vi "RevertVMs.vi"(8 "error in (no error)":errorcluster, 10 "Array":bool[](array[boolean])=[TRUE, TRUE, TRUE, TRUE, TRUE, TRUE, TRUE, TRUE]) -> (0 "error out":errorcluster)   [LabVIEW 2013]
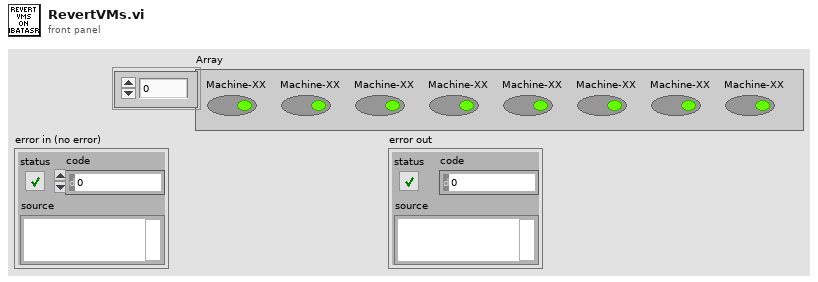
[diagram p1: front panel]
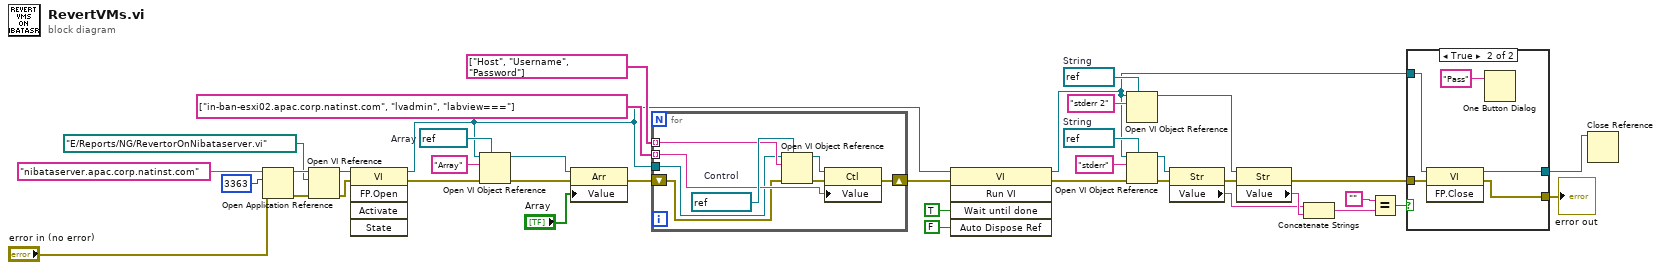
[diagram p0: block diagram]
diagram:
  w18 = refnum<vi> refnum  # String
  w23 = refnum<vi> refnum  # String
  w34 = refnum<vi> refnum  # Array
  n1 = Open Application Reference(8:"error in (no error)", 10:u16 3363 ("port number or service name (3363)"), 11:"nibataserver.apac.corp.natinst.com" ("machine name (\"\":  open local reference)")) -> (0:w37:errorcluster, 3:w36:refnum<vi>)  [unwired: 1 in]
  n2 = Open VI Reference(application reference (local)=w36, vi path=path "E:/Reports/NG/RevertorOnNibataserver.vi", error in (no error)=w37) -> (vi reference=w35:refnum<vi>, error out=w4:errorcluster)  [unwired: 3 in]
  n3 = invoke class="VI" method="FP.Open"(reference=w35, error in=w4) -> (reference out=w6:refnum<vi>, error out=w7:errorcluster)  [unwired: 3 in, 3 out]
  n4 = Open VI Object Reference(7:w34, 8:w7, 10:"Array" ("Text.Text"), 11:w6) -> (0:w32:errorcluster, 3:w33:refnum<vi>)
  n5 = property class="Arr"(reference=w33, error in=w32, "Value"="Array") -> (error out=w26:errorcluster)  [unwired: 1 out]
  n6 = for {
    tunnel: string[] ["Host", "Username", "Password"] -> [w45] mode=indexing
    tunnel: string[] ["in-ban-esxi02.apac.corp.natinst.com", "lvadmin", "labview==="] -> [w44] mode=indexing
    shift-right: [w42] -> w12
    shift-left: w26 -> [w41]
    tunnel: w6 -> [w40]
    w47 = refnum<vi> refnum  # Control
    n7 = Open VI Object Reference(7:w47, 8:w41, 10:w45, 11:w40) -> (0:w43:errorcluster, 3:w46:refnum<vi>)
    n8 = property class="Ctl"(reference=w46, error in=w43, "Value"=w44) -> (error out=w42:errorcluster)  [unwired: 1 out]
  }
  n9 = invoke class="VI" method="Run VI"(reference=w6, error in=w12, "Wait until done"=TRUE ("Wait Until Done"), "Auto Dispose Ref"=FALSE ("Auto Dispose Reference")) -> (reference out=w5:refnum<vi>, error out=w11:errorcluster)  [unwired: 1 in, 3 out]
  n10 = Open VI Object Reference(7:w18, 10:"stderr 2" ("name/order"), 11:w5) -> (3:w20:refnum<vi>)  [unwired: 1 in, 1 out]
  n11 = Open VI Object Reference(7:w23, 8:w11, 10:"stderr" ("name/order"), 11:w5) -> (0:w10:errorcluster, 3:w21:refnum<vi>)
  n12 = property class="Str"(reference=w21, error in=w10) -> (error out=w9:errorcluster, "Value"=w16:string)  [unwired: 1 out]
  n13 = property class="Str"(reference=w20, error in=w9) -> (error out=w8:errorcluster, "Value"=w17:string)  [unwired: 1 out]
  n14 = Concatenate Strings(w16, w17) -> (w15:string)
  n15 = Equal?(x="", y=w15) -> (x = y?=w13:bool)
  n16 = case shown="True" w13 {
    tunnel: w8 -> [w48 w52]
    tunnel: w5 -> [w49 w53]
    tunnel: [w49 w51] -> w2
    tunnel: [w48 w50] -> w1
    frame False {
    }
    frame True {
      n17 = invoke class="VI" method="FP.Close"(reference=w53, error in=w52) -> (reference out=w51:refnum<vi>, error out=w50:errorcluster)  [unwired: 1 in, 1 out]
      n18 = One Button Dialog(message="Pass") -> ()  [unwired: 1 in, 1 out]
    }
  }
  "error out" <- w1
  n19 = Close Reference(reference=w2) -> ()  [unwired: 1 in, 1 out]
